vi "Build RT Data Cluster.vi"(0 "Device Reference in":T1 format="%.0x", 2 "RT Data in":T2={"Device ref"=0, "Scan Period (uSec)"=10000, "Device Channels"={"Status"={"BD Refs"=[], "Length"=0, "FIFO Index"=0, "Data"=[]}, "Command"={"BD Refs"=[], "Data"=[], "Length"=0, "FIFO Index"=0}}, "Local Chassis"=[], "EtherCAT Masters"=[], "Async"={"Status"=refnum, "Command"=refnum, "Input FIFO"=refnum, "Input FIFO buffer"=[], "Output FIFO"=refnum, "Output FIFO buffer"=[], "Async VI Ref"=refnum}, "ECAT Reconfig"={"Reconfig Module Found"=FALSE, "VI Ref"=refnum, "Status"=refnum}, "Device Error"={"status"=FALSE, "code"=0, "source"=""}, "DeviceName"="", "PCLSync?"=FALSE} {"Device Channels"."Status"."BD Refs"."Data Reference" format="%.0x"; "Device Channels"."Command"."BD Refs"."Data Reference" format="%.0x"; "Local Chassis"."FPGA"."VS ref" format="%.0x"; "Local Chassis"."RSI Modules"."VS ref" format="%.0x"; "Local Chassis"."VS ref" format="%.0x"; "Device ref" format="%.0x"; "EtherCAT Masters"."DS402 Drive ECAT Slaves"."VS ref" format="%.0x"; "EtherCAT Masters"."REM IO ECAT Slaves"."VS ref" format="%.0x"; "EtherCAT Masters"."Generic EtherCAT Slaves"."VS ref" format="%.0x"; "EtherCAT Masters"."VS ref" format="%.0x"; "EtherCAT Masters"."EtherCAT Slaves"."FPGA"."VS ref" format="%.0x"; "EtherCAT Masters"."EtherCAT Slaves"."RSI Modules"."VS ref" format="%.0x"; "EtherCAT Masters"."EtherCAT Slaves"."VS ref" format="%.0x"}, 3 "error in":errorcluster) -> (7 "RT Data out":T2={"Device ref"=0, "Scan Period (uSec)"=10000, "Device Channels"={"Status"={"BD Refs"=[], "Length"=0, "FIFO Index"=0, "Data"=[]}, "Command"={"BD Refs"=[], "Data"=[], "Length"=0, "FIFO Index"=0}}, "Local Chassis"=[], "EtherCAT Masters"=[], "Async"={"Status"=refnum, "Command"=refnum, "Input FIFO"=refnum, "Input FIFO buffer"=[], "Output FIFO"=refnum, "Output FIFO buffer"=[], "Async VI Ref"=refnum}, "ECAT Reconfig"={"Reconfig Module Found"=FALSE, "VI Ref"=refnum, "Status"=refnum}, "Device Error"={"status"=FALSE, "code"=0, "source"=""}, "DeviceName"="", "PCLSync?"=FALSE} {"Device Channels"."Status"."BD Refs"."Data Reference" format="%.0x"; "Device Channels"."Command"."BD Refs"."Data Reference" format="%.0x"; "Local Chassis"."FPGA"."VS ref" format="%.0x"; "Local Chassis"."RSI Modules"."VS ref" format="%.0x"; "Local Chassis"."VS ref" format="%.0x"; "Device ref" format="%.0x"; "EtherCAT Masters"."DS402 Drive ECAT Slaves"."VS ref" format="%.0x"; "EtherCAT Masters"."REM IO ECAT Slaves"."VS ref" format="%.0x"; "EtherCAT Masters"."Generic EtherCAT Slaves"."VS ref" format="%.0x"; "EtherCAT Masters"."VS ref" format="%.0x"; "EtherCAT Masters"."EtherCAT Slaves"."FPGA"."VS ref" format="%.0x"; "EtherCAT Masters"."EtherCAT Slaves"."RSI Modules"."VS ref" format="%.0x"; "EtherCAT Masters"."EtherCAT Slaves"."VS ref" format="%.0x"})   [LabVIEW 2016, in "Scan Engine Custom Device.lvlib"]
uses:
  Scan Engine Custom Device.lvlib
  Type Defs/RT Data.ctl
  <vilib>/NI Veristand/Custom Device API/Custom Device Item Ref.ctl
  Type Defs/Device Channels.ctl
  Type Defs/Output Data.ctl
  <vilib>/NI Veristand/Custom Device API/Block Data Reference.ctl
  <vilib>/NI Veristand/Custom Device API/Data Reference.ctl
  Type Defs/Input Data.ctl
  Type Defs/Local Chassis Data.ctl
  Type Defs/RSI Module Data.ctl
  Type Defs/Open Module IOVs.ctl
  Modules.lvlibp/RSI Module/RSI Module.lvclass
  Modules.lvlibp/RSI Module/Module Models.ctl
  Modules.lvlibp/RSI Module/Channel Type.ctl
  Type Defs/Module Config Data.ctl
  Type Defs/Mixed IO.ctl
  Type Defs/FPGA Data.ctl
  Type Defs/UDV Data.ctl
  Type Defs/UDV Data Type.ctl
  Type Defs/FXP Config.ctl
  Type Defs/Mod Size Indexes.ctl
  Type Defs/EtherCAT Master Data.ctl
  Type Defs/EtherCAT Slave Data.ctl
  Type Defs/Generic ECAT Slave RT-Data-Array.ctl
  Type Defs/Generic ECAT Slave Data Cluster.ctl
  Type Defs/Generic ECAT Slave IOV Cluster.ctl
  Type Defs/REM IO ECAT Slave RT-Data-Array.ctl
  Type Defs/REM IO ECAT Slave Data Cluster.ctl
  Type Defs/REM IO ECAT Slave IOV Cluster.ctl
  Type Defs/DS402 Drive ECAT Slave RT-Data-Array.ctl
  Type Defs/DS402 Drive ECAT Slave Data Cluster.ctl
  Type Defs/DS402 Drive ECAT Slave IOV Cluster.ctl
  Type Defs/DS402 Drive ECAT Slave Action IOV Cluster.ctl
  DS402 StateMachine/Library/controls/state.ctl
  Type Defs/Async Data.ctl
  Type Defs/Async Status.ctl
  Type Defs/Async State.ctl
  Type Defs/Async Command.ctl
  Type Defs/ECAT Reconfig Data.ctl
  Type Defs/ECAT Reconfig Status.ctl
  Type Defs/ECAT Reconfig State.ctl
  Type Defs/Data Ref FGV Command.ctl
  <vilib>/NIScanEngine/ConfigurableFaults/Fault Desc Control.ctl
  Globals/Property Strings.vi
  Globals/RT Globals.vi
  Globals/String Constants.vi
  <vilib>/NI Veristand/Custom Device API/Get Item Property (U16).vi
  <vilib>/NI Veristand/Custom Device API/Get Item Property (String).vi
  <vilib>/NI Veristand/Custom Device API/Get Item Property (U32).vi
  <vilib>/NI Veristand/Custom Device API/Custom Device API.lvlib
  <vilib>/NI Veristand/Custom Device Tools/Custom Device Utility Library/Custom Device Utility Library.lvlib
  <vilib>/NIScanEngine/ConfigurableFaults/Config Faults.lvlib
  DS402 StateMachine/Library/DS402.lvlib
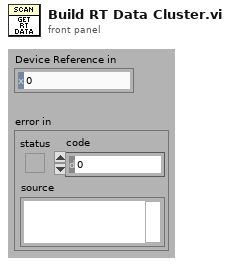
[diagram p1: front panel]
types:
  T1 = typedef "Custom Device API.lvlib/Custom Device Item Ref.ctl" = u64
  T2 = typedef "Scan Engine Custom Device.lvlib/RT Data.ctl" = cluster{"Device ref":T1, "Scan Period (uSec)":u32, "Device Channels":T3, "Local Chassis":T8[], "EtherCAT Masters":T20[], "Async":T33, "ECAT Reconfig":T34, "Device Error":errorcluster, "DeviceName":string, "PCLSync?":bool}
  T3 = typedef "Scan Engine Custom Device.lvlib/Device Channels.ctl" = cluster{"Status":T4, "Command":T7}
  T4 = typedef "Scan Engine Custom Device.lvlib/Output Data.ctl" = cluster{"BD Refs":T5[], "Length":i32, "FIFO Index":i32, "Data":dbl[]}
  T5 = typedef "Custom Device API.lvlib/Block Data Reference.ctl" = cluster{"Data Reference":T6, "Offset":u64, "Length":u64}
  T6 = typedef "Custom Device API.lvlib/Data Reference.ctl" = i32
  T7 = typedef "Scan Engine Custom Device.lvlib/Input Data.ctl" = cluster{"BD Refs":T5[], "Data":dbl[], "Length":i32, "FIFO Index":i32}
  T8 = typedef "Scan Engine Custom Device.lvlib/Local Chassis Data.ctl" = cluster{"VS ref":T1, "RSI Modules":T9[], "FPGA":T15[], "Input Mod Size Idxs":T19, "Output Modules":i32[], "MixedIO Mod Size Idxs":T19}
  T9 = typedef "Scan Engine Custom Device.lvlib/RSI Module Data.ctl" = cluster{"VS ref":T1, "IOV ref":refnum<k21>, "Open Mod refs":T10, "Module DVR":refnum<data-value>, "Slot":u32, "Model":T11, "Channel Type":T12, "EtherCAT?":bool, "CDInput Data":T7, "CDOutput Data":T4, "Module Config Data":T13, "Mixed IO":T14}
  T10 = typedef "Scan Engine Custom Device.lvlib/Open Module IOVs.ctl" = cluster{"Analog Read":refnum<k21>, "Digital Read":refnum<k21>, "Analog Write":refnum<k21>, "Digital Write":refnum<k21>}
  T11 = typedef "Modules.lvlibp/RSI Module.lvclass/Module Models.ctl" = enum16{"Empty", "NI 9201", "NI 9203", "NI 9205", "NI 9206", "NI 9207", "NI 9208", "NI 9211", "NI 9212", "NI 9213", "NI 9214", "NI 9215", "NI 9217", "NI 9219", "NI 9220", "NI 9221", "NI 9222", "NI 9223", "NI 9225", "NI 9227", "NI 9229", "NI 9233", "NI 9234", "NI 9235", "NI 9236", "NI 9237", "NI 9239", "NI 9242", "NI 9244", "NI 9263", "NI 9264", "NI 9265", "NI 9269", "NI 9375", "NI 9401", "NI 9402", "NI 9403", "NI 9411", "NI 9421", "NI 9422", "NI 9423", "NI 9425", "NI 9426", "NI 9435", "NI 9437", "NI 9472", "NI 9474", "NI 9475", "NI 9476", "NI 9477", "NI 9478", "NI 9481", "NI 9482", "NI 9485"}
  T12 = typedef "Modules.lvlibp/RSI Module.lvclass/Channel Type.ctl" = enum16{"Analog", "Digital"}
  T13 = typedef "Scan Engine Custom Device.lvlib/Module Config Data.ctl" = cluster{"Configurable?":bool, "Config Block Data Refs":T5[], "Config Data DVR":refnum<data-value>, "Previous Values":dbl[], "Local Reconfig VI Ref":refnum<vi>}
  T14 = typedef "Scan Engine Custom Device.lvlib/Mixed IO.ctl" = cluster{"Input Channel Indices":i32[], "Input Buffer":dbl[]}
  T15 = typedef "Scan Engine Custom Device.lvlib/FPGA Data.ctl" = cluster{"VS ref":T1, "IOV ref":refnum<k21>, "FPGA Target":enum16{"Local", "EtherCAT"}, "Product Code":u32, "Bitfile Signature":string, "Bitfile Path (RT)":path, "FPGA Session":u32, "Input Data":T7, "Output Data":T4, "UDVs":cluster{"From FPGA":T16[], "To FPGA":T16[]}}
  T16 = typedef "Scan Engine Custom Device.lvlib/UDV Data.ctl" = cluster{"VS ref":T1, "IOV Ref":refnum<k21>, "Name":string, "UDV Data Type":T17, "Supported Type?":bool, "FXP Config":T18, "FXP VI Ref":refnum<vi>}
  T17 = typedef "Scan Engine Custom Device.lvlib/UDV Data Type.ctl" = enum16{"Boolean", "Fixed Point", "Int8", "Int16", "Int32", "Int64", "U32 Bit Field", "UInt8", "UInt16", "UInt32", "UInt64", "Other"}
  T18 = typedef "Scan Engine Custom Device.lvlib/FXP Config.ctl" = cluster{"signed":bool, "size":u32, "integersize":i32}
  T19 = typedef "Scan Engine Custom Device.lvlib/Mod Size Indexes.ctl" = cluster{"4":i32[], "8":i32[], "16":i32[], "32":i32[], "other":i32[]}
  T20 = typedef "Scan Engine Custom Device.lvlib/EtherCAT Master Data.ctl" = cluster{"VS ref":T1, "IOV ref":refnum<k21>, "Master ID":u32, "Cyclic Data Bandwidth":u32, "EtherCAT Slaves":T21[], "Generic EtherCAT Slaves":T22, "REM IO ECAT Slaves":T25, "DS402 Drive ECAT Slaves":T28}
  T21 = typedef "Scan Engine Custom Device.lvlib/EtherCAT Slave Data.ctl" = cluster{"VS ref":T1, "IOV ref":refnum<k21>, "Position Address":u16, "RSI Modules":T9[], "FPGA":T15[], "Input Mod Size Idxs":T19, "Output Modules":i32[], "MixedIO Mod Size Idxs":T19}
  T22 = typedef "Scan Engine Custom Device.lvlib/Generic ECAT Slave RT-Data-Array.ctl" = T23[]
  T23 = typedef "Scan Engine Custom Device.lvlib/Generic ECAT Slave Data Cluster.ctl" = cluster{"VS ref":T1, "IOV ref":refnum<k21>, "Position Address":u16, "I/O Imput Vars ":T24[], "I/O Output Vars":T24[], "I/O Input Data":T7, "I/O Output Data":T4}
  T24 = typedef "Scan Engine Custom Device.lvlib/Generic ECAT Slave IOV Cluster.ctl" = cluster{"VS ref":T1, "IOV Ref":refnum<k21>, "Name":string, "UDV Data Type":T17}
  T25 = typedef "Scan Engine Custom Device.lvlib/REM IO ECAT Slave RT-Data-Array.ctl" = T26[]
  T26 = typedef "Scan Engine Custom Device.lvlib/REM IO ECAT Slave Data Cluster.ctl" = cluster{"VS ref":T1, "IOV ref":refnum<k21>, "Position Address":u16, "I/O Imput Vars ":T27[], "I/O Output Vars":T27[], "I/O Input Data":T7, "I/O Output Data":T4}
  T27 = typedef "Scan Engine Custom Device.lvlib/REM IO ECAT Slave IOV Cluster.ctl" = cluster{"VS ref":T1, "IOV Ref":refnum<k21>, "Name":string, "UDV Data Type":T17, "Scaling Factor":dbl}
  T28 = typedef "DS402 Drive ECAT Slave RT-Data-Array.ctl" = T29[]
  T29 = typedef "Scan Engine Custom Device.lvlib/DS402 Drive ECAT Slave Data Cluster.ctl" = cluster{"VS ref":T1, "IOV ref":refnum<k21>, "Position Address":u16, "I/O Input Vars ":T30[], "I/O Output Vars":T30[], "I/O Input Data":T7, "I/O Output Data":T4, "DS402 IOV":T31}
  T30 = typedef "Scan Engine Custom Device.lvlib/DS402 Drive ECAT Slave IOV Cluster.ctl" = cluster{"VS ref":T1, "IOV Ref":refnum<k21>, "Name":string, "UDV Data Type":T17, "Scaling Factor":dbl, "IOV":bool, "VS data Index":i32}
  T31 = typedef "Scan Engine Custom Device.lvlib/DS402 Drive ECAT Slave Action IOV Cluster.ctl" = cluster{"Control Word":refnum<k21>, "Status Word":refnum<k21>, "Input Offset":i32, "Output Offset":i32, "State":T32}
  T32 = typedef "Scan Engine Custom Device.lvlib/DS402.lvlib/state.ctl" = enum16{"Init", "Not Ready to Switch On", "Read Status Word", "Switch on disabled", "Ready to switch on", "Switched on", "Operation enabled", "Fault", "Fault reaction active", "Quick stop active", "Shutdown - Bad State", "Shutdown - Error", "Shutdown - Normal", "Shutdown - Fault"}
  T33 = typedef "Scan Engine Custom Device.lvlib/Async Data.ctl" = cluster{"Status":refnum<queue>, "Command":refnum<queue>, "Input FIFO":refnum<k33>, "Input FIFO buffer":dbl[], "Output FIFO":refnum<k33>, "Output FIFO buffer":dbl[], "Async VI Ref":refnum<vi>}
  T34 = typedef "Scan Engine Custom Device.lvlib/ECAT Reconfig Data.ctl" = cluster{"Reconfig Module Found":bool, "VI Ref":refnum<vi>, "Status":refnum<queue>}
  T35 = typedef "Config Faults.lvlib/Fault Desc Control.ctl" = cluster{"code":i32, "level or level before threshold":i32, "occurrence threshold":u32, "time window in seconds":u32, "level after threshold":i32}
  T36 = typedef "Scan Engine Custom Device.lvlib/Data Ref FGV Command.ctl" = enum16{"Intialize", "Get", "Update"}
  T37 = typedef "Fault.ctl" = cluster{"code":i32, "level":i32, "first reported time":timestamp, "number reported":u32}
  T38 = typedef "Custom Device API.lvlib/Custom Device Channel.ctl" = cluster{"Type":T39, "Units":string, "Default Value":dbl, "Faultable":bool, "Scalable":bool}
  T39 = typedef "Custom Device API.lvlib/Custom Device Channel Type.ctl" = enum16{"Input", "Output"}
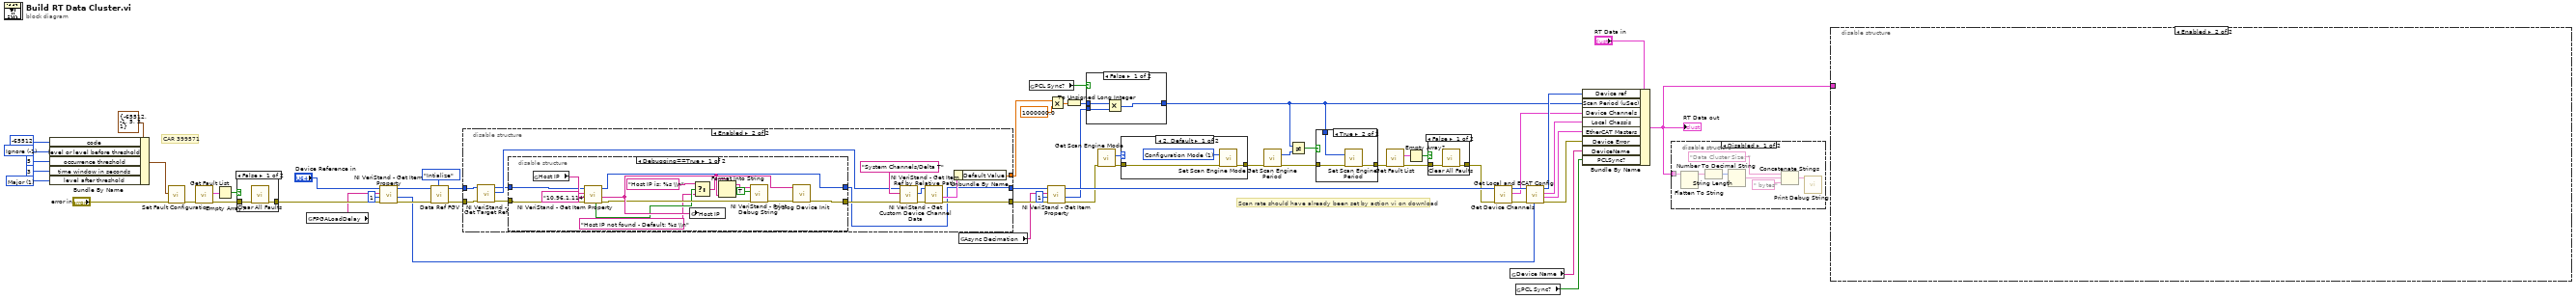
[diagram p0: block diagram]
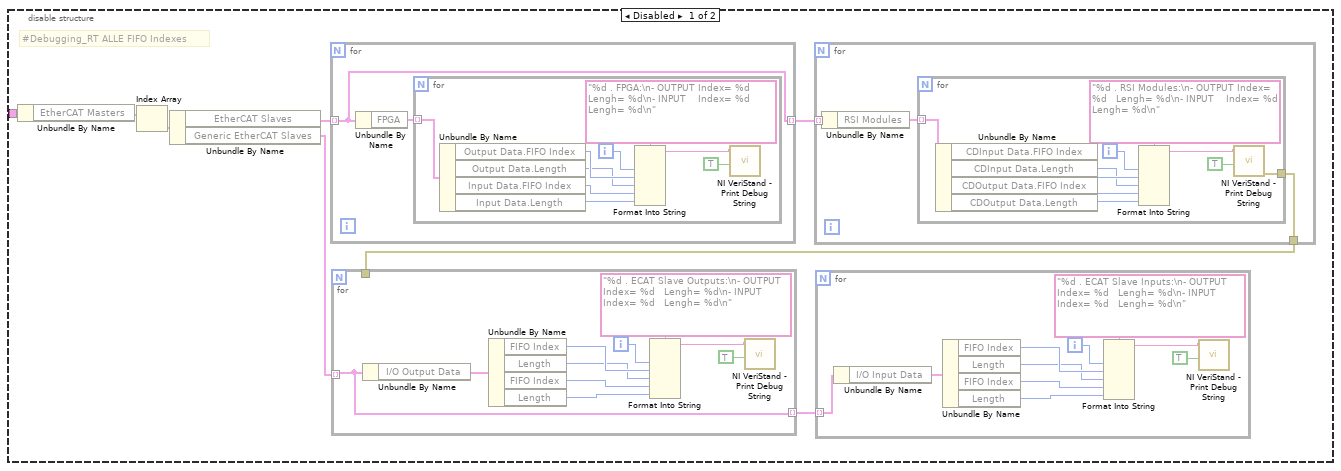
[diagram p2: hidden frame]
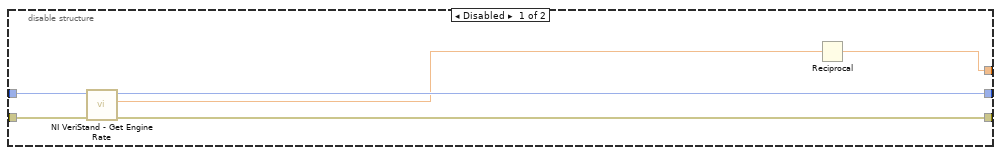
[diagram p9: hidden frame]
diagram:
  w14 = -1 items=["Ignore"=-1, "Minor"=0, "Major"=1] ("level or level before threshold")
  w17 = 1 items=["Ignore"=-1, "Minor"=0, "Major"=1] ("level after threshold")
  # "CAR 399571"
  # "Scan rate should have already been set by action vi on download"
  n1 = Bundle By Name(cluster=T35 {"code"=-65512, "level or level before threshold"=-1, "occurrence threshold"=5, "time window in seconds"=3, "level after threshold"=1} ("fault configuration"), "code"=-65512, "level or level before threshold"=w14, "occurrence threshold"=u32 5, "time window in seconds"=u32 3, "level after threshold"=w17) -> (w18:T35)
  n2 = call <vilib>:"Set Fault Configuration.vi"("error in (no error)"="error in", "fault configuration"=w18) -> ("error out"=w12:errorcluster)  [unwired: 7 in]
  n3 = call <vilib>:"Get Fault List.vi"("error in (no error)"=w12) -> ("error out"=w23:errorcluster, "fault list"=w21:T37[])  [unwired: 9 in]
  n4 = Empty Array?(array=w21) -> (empty?=w22:bool)
  n5 = case shown="False" w22 {
    tunnel: w23 -> [w59 w60]
    tunnel: [w58 w60] -> w20
    frame False {
      n6 = call <vilib>:"Clear All Faults.vi"("error in (no error)"=w59) -> ("error out"=w58:errorcluster)  [unwired: 10 in]
    }
    frame True {
    }
  }
  n7 = global read "Property Strings.vi" "FPGALoadDelay"() -> (w5:string)
  n8 = call-poly <vilib>:"NI VeriStand - Get Item Property.vi"("error in (no error)"=w20, "Default Value"=u16 1, "Property Name"=w5, "Item Ref in"="Device Reference in") -> ("error out"=w8:errorcluster, "Value"=w2:u16, "Item Ref out"=w6:T1)  [unwired: 4 in, 1 out]
  n9 = call "Data Ref FGV.vi"("Command"=Data_Ref_FGV_Command."Intialize", "error in (no error)"=w8, "Device Ref in"=w6) -> ("error out"=w57:errorcluster, "Device Ref out"=w56:T1)  [unwired: 5 in, 2 out]
  n10 = disable-structure shown="Enabled" {
    disable-tunnel: [w61 w74] -> w51
    disable-tunnel: [w66 w73] -> w45
    disable-tunnel: [w65 w67] -> w46
    disable-tunnel: w57 -> [w64 w78]
    disable-tunnel: w56 -> [w63 w79]
    frame Disabled {
      n11 = call <vilib>:"NI VeriStand - Get Engine Rate.vi"("error in (no error)"=w64, "Item Ref in"=w63) -> ("error out"=w66:errorcluster, "Rate (Hz)"=w62:dbl, "Item Ref out"=w65:T1)  [unwired: 7 in]
      n12 = Reciprocal(x=w62) -> (1/x=w61:dbl)
    }
    frame Enabled {
      n13 = call <vilib>:"NI VeriStand - Get Target Ref.vi"("error in"=w78, "Item Ref in"=w79) -> ("error out"=w72:errorcluster, "Target Ref"=w69:T1, "Item Ref out"=w68:T1)  [unwired: 6 in, 1 out]
      n14 = disable-structure shown="Debugging==True" {
        disable-tunnel: w72 -> [w89 w96]
        disable-tunnel: [w91 w96] -> w71
        disable-tunnel: w68 -> [w87 w95]
        disable-tunnel: [w85 w95] -> w67
        frame condition #0 (active) {
          n15 = global read "Property Strings.vi" "Host IP"() -> (w90:string)
          n16 = call-poly <vilib>:"NI VeriStand - Get Item Property.vi"("error in (no error)"=w89, "Default Value"="10.96.1.114", "Property Name"=w90, "Item Ref in"=w87) -> ("error out"=w86:errorcluster, "Value"=w88:string, "Item Ref out"=w85:T1, "Found?"=w83:bool)  [unwired: 4 in]
          n17 = global write "RT Globals.vi" "Host IP"(w88) -> ()
          n18 = Select(t="Host IP is: %s \\n" ("format string"), s=w83, f="Host IP not found - Default: %s \\n" ("format string")) -> (s? t:f=w81:string)
          n19 = Format Into String(format string=w81, w88) -> (resulting string=w94:string)  [unwired: 2 in, 1 out]
          n20 = call <vilib>:"NI VeriStand - Print Debug String.vi"("error in (no error)"=w86, "Add to log file? (T)"=TRUE, "Message"=w94) -> ("error out"=w92:errorcluster)  [unwired: 8 in]
          n21 = call <vilib>:"Syslog Device Init.vi"("error in (no error)"=w92, "Syslog Collector IP Address"=w88) -> ("error out"=w91:errorcluster)  [unwired: 9 in]
        }
        frame condition #1 {
        }
      }
      n22 = call <vilib>:"NI VeriStand - Get Item Ref by Relative Path.vi"("error in"=w71, "Relative Item Path"="System Channels/Delta T", "Section Ref in"=w69) -> ("error out"=w76:errorcluster, "Item Ref"=w77:T1)  [unwired: 5 in, 2 out]
      n23 = call <vilib>:"NI VeriStand - Get Custom Device Channel Data.vi"("error in (no error)"=w76, "Channel Ref in"=w77) -> ("error out"=w73:errorcluster, "Channel"=w75:T38)  [unwired: 4 in, 4 out]
      n24 = Unbundle By Name(w75) -> ("Default Value"=w74:dbl)
    }
  }
  n25 = global read "Property Strings.vi" "Async Decimation"() -> (w43:string)
  n26 = global read "RT Globals.vi" "PCL Sync?"() -> (w40:bool)
  n27 = call-poly <vilib>:"NI VeriStand - Get Item Property.vi"("error in (no error)"=w45, "Default Value"=u32 1, "Property Name"=w43, "Item Ref in"=w46) -> ("error out"=w31:errorcluster, "Value"=w41:u32, "Item Ref out"=w44:T1)  [unwired: 4 in, 1 out]
  n28 = Multiply(x=w51, y=1000000.0) -> (x*y=w25:dbl)
  n29 = To Unsigned Long Integer(number=w25) -> (unsigned 32bit integer=w24:u32)
  n30 = case shown="False" w40 {
    tunnel: w24 -> [w99 w100]
    tunnel: w41 -> [w98 _]
    tunnel: [w97 w100] -> w26
    frame False {
      n31 = Multiply(x=w99, y=w98) -> (x*y=w97:u32)
    }
    frame True {
    }
  }
  n32 = call <vilib>:"Get Scan Engine Mode.vi"("error in (no error)"=w31) -> ("error out"=w33:errorcluster, "mode"=w32:i32)  [unwired: 9 in]
  n33 = case shown="2, Default" w32 {
    tunnel: w33 -> [w102 w104]
    tunnel: [w101 w104] -> w30
    frame 2, Default {
      w103 = 1 items=["Configuration Mode"=1, "Active Mode"=2] ("mode (Active Mode)")
      n34 = call <vilib>:"Set Scan Engine Mode.vi"("mode (Active Mode)"=w103, "error in (no error)"=w102) -> ("error out"=w101:errorcluster)  [unwired: 13 in]
    }
    frame 1 {
    }
  }
  n35 = call <vilib>:"Get Scan Engine Period.vi"("error in (no error)"=w30) -> ("scan period (uSec)"=w29:u32, "error out"=w27:errorcluster)  [unwired: 13 in]
  n36 = Not Equal?(x=w26, y=w29) -> (x != y?=w28:bool)
  n37 = case shown="True" w28 {
    tunnel: [w105 w108] -> w35
    tunnel: w27 -> [w105 w107]
    tunnel: w26 -> [_ w106]
    frame False {
    }
    frame True {
      n38 = call <vilib>:"Set Scan Engine Period.vi"("scan period (uSec)"=w106, "error in (no error)"=w107) -> ("error out"=w108:errorcluster)  [unwired: 13 in]
    }
  }
  n39 = call <vilib>:"Get Fault List.vi"("error in (no error)"=w35) -> ("error out"=w38:errorcluster, "fault list"=w36:T37[])  [unwired: 9 in]
  n40 = Empty Array?(array=w36) -> (empty?=w37:bool)
  n41 = case shown="False" w37 {
    tunnel: w38 -> [w110 w111]
    tunnel: [w109 w111] -> w34
    frame False {
      n42 = call <vilib>:"Clear All Faults.vi"("error in (no error)"=w110) -> ("error out"=w109:errorcluster)  [unwired: 10 in]
    }
    frame True {
    }
  }
  n43 = call "Get Device Channels.vi"("error in"=w34, "Device Reference in"=w44) -> ("error out"=w49:errorcluster, "Device Channels"=w47:T3, "Device Reference out"=w48:T1)  [unwired: 7 in]
  n44 = global read "String Constants.vi" "Device Name"() -> (w10:string)
  n45 = global read "RT Globals.vi" "PCL Sync?"() -> (w9:bool)
  n46 = call "Get Local and ECAT Config.vi"("fpga wait (s)"=w2, "error in (no error)"=w49, "Device Reference in"=w48) -> ("error out"=w3:errorcluster, "ECAT Masters"=w39:T20[], "Local Chassis"=w55:T8[], "Device Reference out"=w53:T1)  [unwired: 5 in]
  n47 = Bundle By Name(cluster="RT Data in", "Device ref"=w53, "Scan Period (uSec)"=w26, "Device Channels"=w47, "Local Chassis"=w55, "EtherCAT Masters"=w39, "Device Error"=w3, "DeviceName"=w10, "PCLSync?"=w9) -> (w1:T2)
  "RT Data out" <- w1
  n48 = disable-structure shown="Disabled" {
    disable-tunnel: w1 -> [w112 _]
    frame Disabled {
      n49 = Flatten To String(anything=w112) -> (data string=w113:string)  [unwired: 3 in, 2 out]
      n50 = String Length(string=w113) -> (length=w115:i32)
      n51 = Number To Decimal String(number=w115) -> (decimal integer string=w116:string)  [unwired: 1 in]
      n52 = Concatenate Strings("Data Cluster Size: " ("string"), w116, " bytes" ("string")) -> (w118:string)
      n53 = call "Print Debug String.vi"("String to write"=w118) -> ()  [unwired: 9 in, 1 out]
    }
    frame Enabled {
    }
  }
  n54 = disable-structure shown="Enabled" {
    disable-tunnel: w1 -> [w126 _]
    frame Disabled {
      # "#Debugging_RT ALLE FIFO Indexes"
      n55 = Unbundle By Name(w126) -> ("EtherCAT Masters"=w125:T20[])
      n56 = Index Array(array=w125) -> (element=w124:T20)  [unwired: 1 in]
      n57 = Unbundle By Name(w124) -> ("EtherCAT Slaves"=w123:T21[], "Generic EtherCAT Slaves"=w121:T22)
      n58 = for {
        tunnel: w123 -> [w160] mode=indexing
        tunnel: [w160] -> w122 mode=indexing
        n59 = Unbundle By Name(w160) -> ("FPGA"=w161:T15[])
        n60 = for {
          tunnel: w161 -> [w170] mode=indexing
          i -> [w166]
          n61 = Unbundle By Name(w170) -> ("Output Data.FIFO Index"=w165:i32, "Output Data.Length"=w164:i32, "Input Data.FIFO Index"=w163:i32, "Input Data.Length"=w162:i32)
          n62 = Format Into String(format string="%d . FPGA:\n- OUTPUT Index= %d   Lengh= %d\n- INPUT    Index= %d   Lengh= %d\n", w166, w165, w164, w163, w162) -> (resulting string=w169:string)  [unwired: 2 in, 1 out]
          n63 = call <vilib>:"NI VeriStand - Print Debug String.vi"("Add to log file? (T)"=TRUE, "Message"=w169) -> ()  [unwired: 9 in, 1 out]
        }
      }
      n64 = for {
        tunnel: w122 -> [w148] mode=indexing
        tunnel: [w147] -> w119
        n65 = Unbundle By Name(w148) -> ("RSI Modules"=w149:T9[])
        n66 = for {
          tunnel: w149 -> [w159] mode=indexing
          tunnel: [w150] -> w147
          i -> [w155]
          n67 = Unbundle By Name(w159) -> ("CDInput Data.FIFO Index"=w154:i32, "CDInput Data.Length"=w153:i32, "CDOutput Data.FIFO Index"=w152:i32, "CDOutput Data.Length"=w151:i32)
          n68 = Format Into String(format string="%d . RSI Modules:\n- OUTPUT Index= %d   Lengh= %d\n- INPUT    Index= %d   Lengh= %d\n", w155, w154, w153, w152, w151) -> (resulting string=w158:string)  [unwired: 2 in, 1 out]
          n69 = call <vilib>:"NI VeriStand - Print Debug String.vi"("Add to log file? (T)"=TRUE, "Message"=w158) -> ("error out"=w150:errorcluster)  [unwired: 9 in]
        }
      }
      n70 = for {
        tunnel: w121 -> [w137] mode=indexing
        tunnel: [w137] -> w120 mode=indexing
        tunnel: w119 -> [_]
        i -> [w143]
        n71 = Unbundle By Name(w137) -> ("I/O Output Data"=w138:T4)
        n72 = Unbundle By Name(w138) -> ("FIFO Index"=w142:i32, "Length"=w141:i32, "FIFO Index"=w140:i32, "Length"=w139:i32)
        n73 = Format Into String(format string="%d . ECAT Slave Outputs:\n- OUTPUT Index= %d   Lengh= %d\n- INPUT    Index= %d   Lengh= %d\n", w143, w142, w141, w140, w139) -> (resulting string=w146:string)  [unwired: 2 in, 1 out]
        n74 = call <vilib>:"NI VeriStand - Print Debug String.vi"("Add to log file? (T)"=TRUE, "Message"=w146) -> ()  [unwired: 9 in, 1 out]
      }
      n75 = for {
        tunnel: w120 -> [w127] mode=indexing
        i -> [w133]
        n76 = Unbundle By Name(w127) -> ("I/O Input Data"=w128:T7)
        n77 = Unbundle By Name(w128) -> ("FIFO Index"=w132:i32, "Length"=w131:i32, "FIFO Index"=w130:i32, "Length"=w129:i32)
        n78 = Format Into String(format string="%d . ECAT Slave Inputs:\n- OUTPUT Index= %d   Lengh= %d\n- INPUT    Index= %d   Lengh= %d\n", w133, w132, w131, w130, w129) -> (resulting string=w136:string)  [unwired: 2 in, 1 out]
        n79 = call <vilib>:"NI VeriStand - Print Debug String.vi"("Add to log file? (T)"=TRUE, "Message"=w136) -> ()  [unwired: 9 in, 1 out]
      }
    }
    frame Enabled {
    }
  }
